vi "Ramp_SubVI.vi"(0 "Enum":enum16{"linear", "power"}(ring), 3 "index":i32, 4 "step":dbl, 5 "end":dbl, 6 "start":dbl) -> (1 "Stop?":bool, 2 "Numeric":dbl)   [LabVIEW 2019]
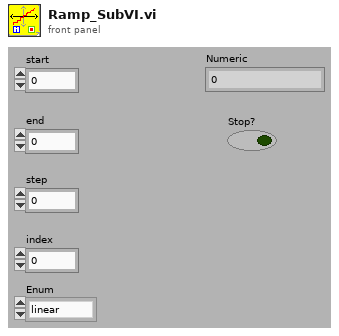
[diagram p1: front panel]
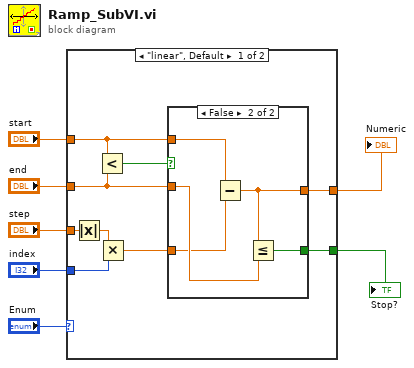
[diagram p0: block diagram]
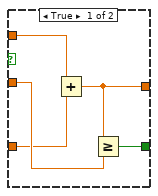
[diagram p2: hidden frame]
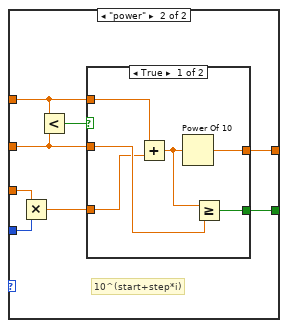
[diagram p3: hidden frame]
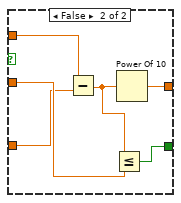
[diagram p4: hidden frame]
diagram:
  n1 = case shown="\"linear\", Default" "Enum" {
    tunnel: "end" -> [w16 w34]
    tunnel: "start" -> [w15 w33]
    tunnel: [w14 w32] -> w5
    tunnel: "step" -> [w11 w29]
    tunnel: "index" -> [w10 w28]
    tunnel: [w12 w30] -> w2
    frame "linear", Default {
      n2 = Absolute Value(x=w11) -> (abs(x)=w8:dbl)
      n3 = Less?(x=w15, y=w16) -> (x < y?=w13:bool)
      n4 = Multiply(x=w8, y=w10) -> (x*y=w9:dbl)
      n5 = case shown="False" w13 {
        tunnel: w15 -> [w21 w26]
        tunnel: [w20 w25] -> w12
        tunnel: w16 -> [w19 w24]
        tunnel: [w18 w23] -> w14
        tunnel: w9 -> [w17 w22]
        frame True {
          n6 = Add(x=w21, y=w17) -> (x+y=w20:dbl)
          n7 = Greater Or Equal?(x=w20, y=w19) -> (x >= y?=w18:bool)
        }
        frame False {
          n8 = Subtract(x=w26, y=w22) -> (x-y=w25:dbl)
          n9 = Less Or Equal?(x=w25, y=w24) -> (x <= y?=w23:bool)
        }
      }
    }
    frame "power" {
      # "10^(start+step*i)"
      n10 = Multiply(x=w29, y=w28) -> (x*y=w27:dbl)
      n11 = Less?(x=w33, y=w34) -> (x < y?=w31:bool)
      n12 = case shown="True" w31 {
        tunnel: w33 -> [w40 w46]
        tunnel: [w36 w42] -> w30
        tunnel: w34 -> [w39 w45]
        tunnel: [w38 w44] -> w32
        tunnel: w27 -> [w37 w43]
        frame True {
          n13 = Add(x=w40, y=w37) -> (x+y=w35:dbl)
          n14 = Power Of 10(x=w35) -> (10^x=w36:dbl)
          n15 = Greater Or Equal?(x=w35, y=w39) -> (x >= y?=w38:bool)
        }
        frame False {
          n16 = Subtract(x=w46, y=w43) -> (x-y=w41:dbl)
          n17 = Less Or Equal?(x=w41, y=w45) -> (x <= y?=w44:bool)
          n18 = Power Of 10(x=w41) -> (10^x=w42:dbl)
        }
      }
    }
  }
  "Numeric" <- w2
  "Stop?" <- w5
